vi "BuildProbabilities.vi"(9 "z":dbl[](array[numeric]), 10 "y":dbl[](array[numeric]), 11 "x":dbl[](array[numeric])) -> (3 "xyz":dbl[](array[numeric]))   [LabVIEW 2014]
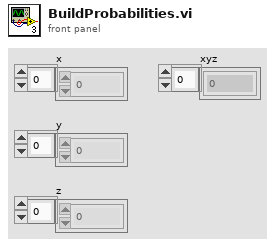
[diagram p1: front panel]
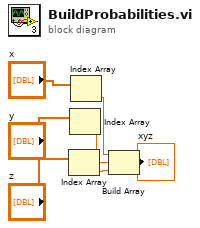
[diagram p0: block diagram]
diagram:
  n1 = Index Array(array="z") -> (element=w4:dbl)  [unwired: 1 in]
  n2 = Index Array(array="y") -> (element=w5:dbl)  [unwired: 1 in]
  n3 = Index Array(array="x") -> (element=w6:dbl)  [unwired: 1 in]
  n4 = Build Array(w6, w5, w4) -> (→"xyz":dbl[])
